vi "Initialize Tree.vi"(8 "error in (no error)":errorcluster, 11 "Configuration":T1) -> (0 "error out":errorcluster, 3 "Configuration Out":T1={"Data Tree Ref"=refnum, "FP Ref"=refnum, "Column Data Type"=[], "Search Clones Up To"=100, "SortOptions"={"Col.pri"=0, "RevDir.pri"=FALSE, "Col.sec"=0, "RevDir.sec"=FALSE}, "Group/Flat (0:group)"=FALSE, "CollapsedNodes"=[], "Show/Hide Cols"=[], "Filtered Paths"=[], "View"=enum."Group By Library", "File Extension Filters"=[], "Filter Global VIs"=FALSE, "Shared"=refnum, "Active Filters"=refnum, "Refresh Rate (ms)"=2000, "App Instance Ring Ref"=refnum, "Processing Q"=refnum, "VI Ref"=refnum})   [LabVIEW 2013, in "LVTM.lvlib"]
uses:
  LVTM.lvlib
  Controls_LVTM/LVTM_Config_Info.ctl
  Controls_LVTM/View.ctl
  Controls_LVTM/SharedDataDVR.ctl
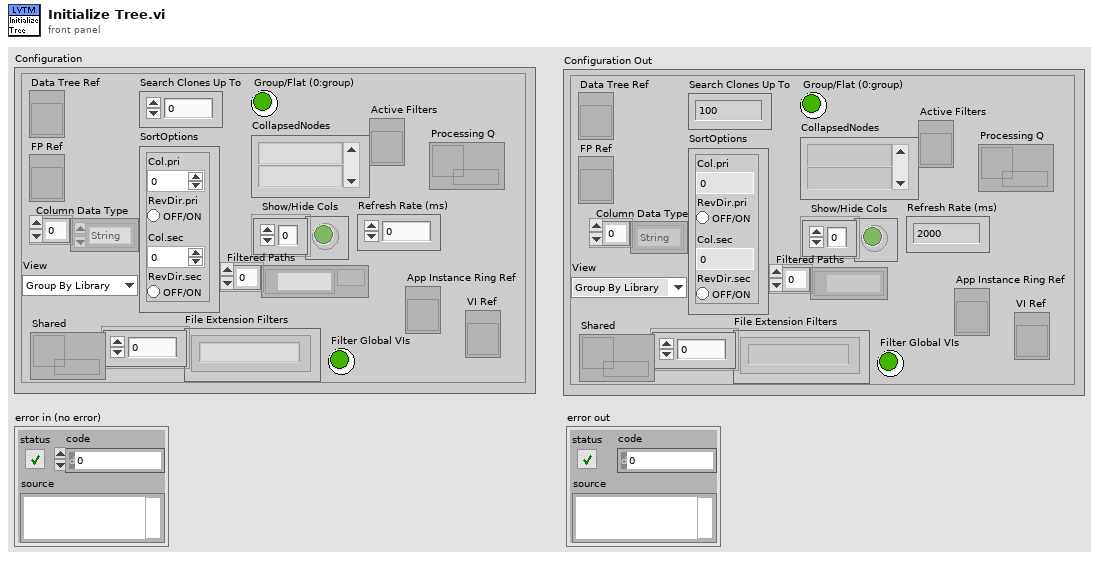
[diagram p1: front panel]
types:
  T1 = typedef "LVTM.lvlib/LVTM_Config_Info.ctl" = cluster{"Data Tree Ref":refnum<vi>, "FP Ref":refnum<vi>, "Column Data Type":enum16{"String", "Numeric"}[], "Search Clones Up To":i32, "SortOptions":cluster{"Col.pri":i32, "RevDir.pri":bool, "Col.sec":i32, "RevDir.sec":bool}, "Group/Flat (0:group)":bool, "CollapsedNodes":string[], "Show/Hide Cols":bool[], "Filtered Paths":path[], "View":T2, "File Extension Filters":string[], "Filter Global VIs":bool, "Shared":refnum<data-value>, "Active Filters":refnum<vi>, "Refresh Rate (ms)":i32, "App Instance Ring Ref":refnum<vi>, "Processing Q":refnum<queue>, "VI Ref":refnum<vi>}
  T2 = typedef "LVTM.lvlib/View.ctl" = enum16{"Group By Library", "Group By Folder", "Flat List"}
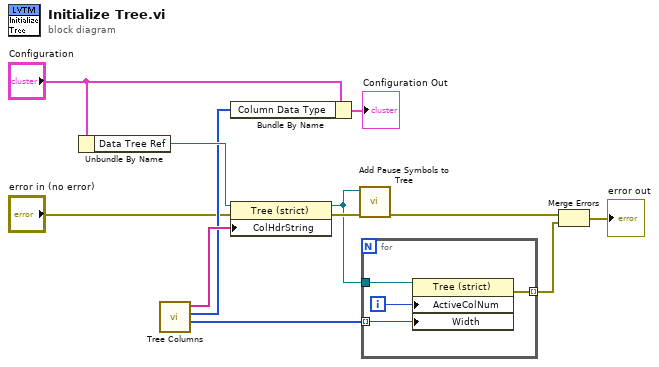
[diagram p0: block diagram]
diagram:
  n1 = Unbundle By Name("Configuration") -> ("Data Tree Ref"=w11:refnum<vi>)
  n2 = call "Tree Columns.vi"() -> ("Column Widths"=w4:i32[], "Column Data Type"=w2:enum16{"String", "Numeric"}[], "Column Labels"=w3:string[])  [unwired: 8 in, 1 out]
  n3 = Bundle By Name(cluster="Configuration", "Column Data Type"=w2) -> (→"Configuration Out":T1)
  n4 = property on="Property Node" class="Tree (strict)"(reference=w11, error in="error in (no error)", "ColHdrString"=w3) -> (reference out=w8:refnum<vi>, error out=w12:errorcluster)
  n5 = call "Add Pause Symbols to Tree.vi"("error in"=w12, "Data Tree Ref"=w8) -> ("error out"=w5:errorcluster)  [unwired: 9 in]
  n6 = for {
    tunnel: w8 -> [w16]
    tunnel: w4 -> [w14] mode=indexing
    tunnel: [w13] -> w6 mode=indexing
    i -> [w15]
    n7 = property on="Property Node" class="Tree (strict)"(reference=w16, "ActiveColNum"=w15, "Width"=w14) -> (error out=w13:errorcluster)  [unwired: 1 in, 1 out]
  }
  n8 = Merge Errors(w5, w6) -> (→"error out":errorcluster)
